vi "_make_3d_data2.vi"(11 "mk3d":T1={"Start(GHz)"=786.0, "Stop(GHz) "=954.0, "Step(GHz) "=8.0, "パス"=path "C:/Documents and Settings/?澤佳?/デスクトップ/data/SISmixer/1108-/110825_O501_164-3-4-B1", "最初のファイル名"="", "取得列 Z"=4, "Text line skip"=0, "リングZ"=0, "リングX"=0, "取得列 X"=0} {"リングX" items=["IF(GHz)", "V(mV)"]; "リングZ" items=["Trx(K)", "I (mA)", "P_PM (dBm)", "P_SP(dBm)", "SBR (dB)", "POUT(dBm/100MHz)", "P-P(dB)"]}) -> (3 "出力ファイル名":string="IV-TRx__matrix_data40_110_110824_O501_164-3-4-B1m.csv.png")   [LabVIEW 2017]
uses:
  <vilib>/Utility/file.llb/Read From Spreadsheet File (string).vi
  <vilib>/Utility/file.llb/Write To Spreadsheet File (DBL).vi
  <vilib>/express/express arith-compare/Formula/XNode/ExpressFormulaBlockNode.xnode
panel:
  out "配列 2":dbl[][](array[numeric])=[[0.0, -0.021515, 0.021133, 0.072174, 0.118256, 0.166397, 0.216446, 0.26619, 0.316162, 0.365219, 0.412979, 0.462189, 0.510864, 0.56633, 0.610428, 0.660324, 0.711594, 0.765305, 0.81337, 0.85968, 0.909805, 0.960464, 1.009, 1.058, 1.125, 1.162, 1.21, 1.26, 1.309, 1.356, 1.412, 1.462, 1.515, 1.567, 1.616, 1.659, 1.711, 1.761, 1.81, 1.858, 1.911, 1.959, 2.009, 2.058, 2.114, 2.159, 2.211, 2.261, 2.316, 2.361, 2.408, 2.456, 2.505, 2.543, 2.576, 2.63, 2.68, 2.75, 2.809, 2.858, 2.912, 2.959, 3.009, 3.063, 3.118, 3.158, 3.208, 3.26, 3.312, 3.358, 3.408, 3.456], [0.0, -2.759, 0.949097, 1.77, 2.716, 3.891, 4.715, 4.971, 5.508, 5.536, 6.039, 6.192, 6.519, 7.303, 7.278, 7.269, 7.129, 7.376, 7.846, 7.675, 7.837, 7.706, 8.182, 8.075, 8.951, 8.67, 8.627, 8.762, 9.293, 9.412, 10.156, 10.516, 10.919, 10.989, 13.586, 11.472, 11.914, 11.996, 12.283, 12.628, 12.357, 12.534, 13.037, 13.245, 12.537, 15.952, 14.566, 14.828, 15.811, 16.809, 17.337, 19.51, 25.082, 46.259, 95.831, 183.994, 262.131, 277.545, 282.7, 286.295, 289.304, 293.353, 297.006, 301.584, 306.857, 311.581, 315.21, 320.633, 325.778, 330.511, 336.539, 341.284], [0.0, -0.024796, 0.014496, 0.070648, 0.117722, 0.16922, 0.21492, 0.268326, 0.313416, 0.36438, 0.413513, 0.462646, 0.50354, 0.561981, 0.611191, 0.662842, 0.711517, 0.765381, 0.815582, 0.861969, 0.909119, 0.95932, 1.012, 1.055, 1.111, 1.16, 1.212, 1.257, 1.312, 1.359, 1.41, 1.46, 1.516, 1.585, 1.615, 1.661, 1.712, 1.76, 1.81, 1.858, 1.912, 1.959, 2.009, 2.056, 2.117, 2.159, 2.211, 2.257, 2.315, 2.36, 2.412, 2.457, 2.506, 2.542, 2.579, 2.621, 2.683, 2.75, 2.807, 2.854, 2.91, 2.96, 3.01, 3.061, 3.119, 3.168, 3.21, 3.26, 3.308, 3.357, 3.409, 3.459], [0.0, -3.03, -0.485229, 2.176, 2.954, 4.175, 4.663, 4.852, 5.463, 5.704, 5.875, 6.094, 6.351, 6.937, 6.775, 7.181, 7.242, 8.023, 7.538, 7.535, 7.892, 7.913, 9.131, 9.052, 7.916, 8.554, 8.661, 8.954, 9.329, 9.561, 10.172, 10.565, 10.916, 11.685, 10.901, 11.368, 11.713, 11.697, 11.792, 12.274, 12.714, 12.448, 12.659, 11.96, 13.339, 14.093, 14.365, 14.911, 15.134, 16.608, 17.584, 19.22, 24.85, 45.2, 92.975, 180.786, 262.372, 277.557, 282.654, 286.032, 289.508, 293.164, 297.324, 301.791, 306.183, 313.147, 315.915, 320.572, 325.543, 331.009, 335.779, 341.519], [0.0, -27.782, -27.509, -29.831, -30.166, -29.882, -28.631, -28.059, -27.897, -27.987, -28.03, -28.065, -27.894, -27.883, -27.792, -27.707, -27.619, -27.792, -27.859, -27.648, -27.37, -27.164, -27.236, -27.394, -27.417, -27.784, -28.542, -29.174, -29.587, -29.571, -29.224, -28.128, -27.366, -26.908, -26.869, -26.719, -26.736, -26.695, -26.838, -26.814, -26.894, -26.348, -26.722, -26.212, -27.382, -27.686, -28.04, -28.527, -29.379, -29.979, -30.586, -31.535, -31.921, -31.348, -31.463, -31.376, -31.686, -30.693, -28.887, -28.036, -28.149, -28.582, -28.835, -28.902, -29.247, -29.316, -29.396, -29.27, -29.234, -29.183, -29.27, -29.233], [0.0, -27.853, -27.485, -29.964, -30.242, -29.717, -28.74, -27.99, -27.882, -28.019, -27.992, -28.197, -27.874, -27.821, -27.809, -27.741, -27.682, -27.792, -27.834, -27.657, -27.449, -27.285, -27.255, -27.421, -27.545, -27.779, -28.486, -29.17, -29.811, -30.056, -29.474, -28.54, -27.809, -27.477, -27.297, -27.124, -27.187, -27.217, -27.343, -27.378, -27.574, -26.883, -27.179, -26.729, -27.946, -28.387, -28.588, -28.94, -29.945, -30.284, -30.987, -31.769, -31.705, -31.834, -31.129, -31.0, -31.339, -30.359, -28.886, -28.164, -28.369, -28.632, -28.643, -28.957, -29.154, -29.248, -29.247, -29.318, -29.311, -29.24, -29.322, -29.566], [0.0, 10000.0, 0.0, 7029.0, 10000.0, 0.0, 8633.0, 0.0, 0.0, 10000.0, 0.0, 7113.0, 0.0, 0.0, 10000.0, 10000.0, 10000.0, 10000.0, 0.0, 10000.0, 10000.0, 7792.0, 10000.0, 10000.0, 7334.0, 0.0, 0.0, 0.0, 4110.0, 1801.0, 3669.0, 2155.0, 1989.0, 1508.0, 2069.0, 2196.0, 1951.0, 1663.0, 1724.0, 1524.0, 1232.0, 1618.0, 1923.0, 1679.0, 1523.0, 1190.0, 1574.0, 2145.0, 1520.0, 2974.0, 2219.0, 3933.0, 0.0, 1800.0, 0.0, 0.0, 0.0, 0.0, 0.0, 7289.0, 4197.0, 10000.0, 0.0, 10000.0, 0.0, 0.0, 0.0, 10000.0, 10000.0, 10000.0, 10000.0, 2710.0], [0.0, 0.0, 0.05, 0.1, 0.15, 0.2, 0.25, 0.3, 0.35, 0.4, 0.45, 0.5, 0.55, 0.6, 0.65, 0.7, 0.75, 0.8, 0.85, 0.9, 0.95, 1.0, 1.05, 1.1, 1.15, 1.2, 1.25, 1.3, 1.35, 1.4, 1.45, 1.5, 1.55, 1.6, 1.65, 1.7, 1.75, 1.8, 1.85, 1.9, 1.95, 2.0, 2.05, 2.1, 2.15, 2.2, 2.25, 2.3, 2.35, 2.4, 2.45, 2.5, 2.55, 2.6, 2.65, 2.7, 2.75, 2.8, 2.85, 2.9, 2.95, 3.0, 3.05, 3.1, 3.15, 3.2, 3.25, 3.3, 3.35, 3.4, 3.45, 3.5]]
  in  "タブ制御器":enum32{"SP ファイル", "YIG関係"}(tab)
  in  "配列 X":T2(array[cluster])=[{"Y label"="IF(GHz)", "Y  range [min:max] "="[3.5:12.5]"}, {"Y label"="V  (mV)", "Y  range [min:max] "="[0:3]"}, {"Y label"="Vg (V)", "Y  range [min:max] "="[0:4]"}, {"Y label"="", "Y  range [min:max] "=""}]
  in  "配列 Z":T3(array[cluster])=[{"Z label"="Trx (K)", "Z  range [min:max] "="[0:500]", "contour  param(start,step,stop) "="200,25,300"}, {"Z label"="I  (mA)", "Z  range [min:max] "="[0:300]", "contour  param(start,step,stop) "="0,10,300"}, {"Z label"="P (dBm)", "Z  range [min:max] "="[-30:-10]", "contour  param(start,step,stop) "="-30,1,-10"}, {"Z label"="P(dBm)", "Z  range [min:max] "="[-60:-40]", "contour  param(start,step,stop) "="-60,5,-40"}, {"Z label"="SBR (dB)", "Z  range [min:max] "="[-2:2]", "contour  param(start,step,stop) "="-3,1,3"}, {"Z label"="Pout (dBm/100MHz)", "Z  range [min:max] "="[-60:-40]", "contour  param(start,step,stop) "="-60,2,-40"}, {"Z label"="PP (dB)", "Z  range [min:max] "="[0:5]", "contour  param(start,step,stop) "="0,1,5"}]
  in  "gnuplotのパス":string="C:\\wintool\\gnuplot\\bin\\wgnuplot.exe  "
  in  "Soption (b:bottom s:surface t:top))":string="sb"
  in  "y  range[min:max]":string="[780:960]"
  in  "y label":string="LO (GHz)"
  out "配列":dbl[][](array[numeric])=[[0.0, 0.0, 0.0, 0.0, 0.0, 0.0, 0.0, 0.0, 0.0, 0.0, 0.0, 0.0, 0.0, 0.0, 0.0, 0.0, 0.0, 0.0, 0.0, 0.0, 0.0, 0.0, 0.0, 0.0, 0.0], [-30.052, -29.746, -29.814, -29.969, -29.665, -29.662, -28.995, -29.934, -30.166, -28.878, -29.619, -29.495, -29.613, -29.184, -28.402, -29.501, -28.588, -28.796, -28.742, -28.754, -28.339, -28.165, -28.518, -27.55, -27.782], [-29.027, -28.715, -29.153, -29.409, -28.957, -29.033, -28.252, -29.414, -29.542, -28.472, -28.837, -28.831, -29.105, -28.292, -27.806, -28.872, -28.1, -28.123, -28.085, -27.916, -27.924, -27.581, -27.997, -27.21, -27.509], [-30.39, -30.323, -30.61, -30.514, -30.678, -30.654, -30.446, -30.508, -30.773, -30.427, -30.544, -30.65, -30.828, -30.482, -30.144, -30.751, -30.552, -30.361, -30.39, -30.146, -30.34, -30.09, -30.3, -29.667, -29.831], [-29.941, -30.022, -30.034, -30.152, -30.317, -30.094, -30.247, -29.872, -30.239, -30.155, -30.317, -30.36, -30.161, -30.262, -30.274, -30.45, -30.369, -30.538, -30.387, -30.182, -30.194, -30.301, -30.351, -30.318, -30.166], [-28.925, -29.309, -29.101, -29.024, -29.103, -29.316, -29.286, -29.285, -29.12, -29.296, -29.419, -29.231, -29.206, -29.34, -29.929, -29.347, -29.672, -29.324, -29.631, -29.465, -29.709, -29.809, -29.655, -29.951, -29.882], [-27.534, -27.559, -27.511, -27.483, -27.798, -27.794, -27.95, -27.71, -27.643, -28.116, -27.783, -28.156, -27.971, -28.202, -28.349, -28.001, -28.379, -28.279, -28.292, -28.389, -28.395, -28.661, -28.371, -28.745, -28.631], [-26.036, -26.401, -26.124, -26.16, -26.51, -26.709, -26.965, -26.46, -26.442, -27.173, -26.796, -26.837, -26.903, -27.301, -27.705, -26.97, -27.513, -27.389, -27.423, -27.39, -27.429, -27.905, -27.423, -28.067, -28.059], [-25.829, -26.185, -25.986, -25.886, -26.231, -26.422, -26.794, -26.247, -26.126, -26.991, -26.688, -26.759, -26.603, -27.026, -27.613, -26.914, -27.266, -27.28, -27.337, -27.27, -27.296, -27.659, -27.438, -27.889, -27.897], [-26.711, -26.496, -26.21, -25.972, -26.228, -26.532, -26.853, -26.326, -26.339, -27.059, -26.765, -26.9, -26.796, -27.158, -27.589, -26.921, -27.433, -27.338, -27.443, -27.274, -27.496, -27.778, -27.462, -28.052, -27.987], [-28.336, -27.383, -26.586, -26.145, -26.328, -26.356, -26.898, -26.354, -26.401, -27.037, -26.97, -27.006, -26.848, -27.248, -27.617, -27.031, -27.525, -27.393, -27.36, -27.493, -27.639, -27.937, -27.571, -28.159, -28.03], [-30.165, -29.108, -27.819, -26.759, -26.475, -26.453, -26.784, -26.296, -26.33, -26.843, -26.885, -26.938, -26.875, -27.147, -27.536, -26.999, -27.437, -27.452, -27.364, -27.453, -27.545, -27.76, -27.662, -28.081, -28.065], [-31.108, -30.641, -29.672, -28.14, -27.396, -26.804, -26.822, -26.039, -25.963, -26.847, -26.635, -26.742, -26.702, -27.062, -27.54, -26.868, -27.324, -27.242, -27.31, -27.289, -27.472, -27.718, -27.466, -27.959, -27.894], [-31.325, -30.996, -30.956, -29.909, -29.093, -27.988, -27.362, -26.275, -25.974, -26.651, -26.392, -26.567, -26.474, -26.867, -27.365, -26.889, -27.282, -27.227, -27.151, -27.316, -27.235, -27.651, -27.325, -28.021, -27.883], [-31.412, -31.069, -31.373, -31.118, -30.681, -29.401, -28.533, -27.065, -26.318, -26.605, -26.309, -26.359, -26.346, -26.885, -27.277, -26.875, -27.221, -27.212, -27.162, -27.382, -27.401, -27.743, -27.438, -28.015, -27.792], [-30.967, -30.611, -31.231, -31.187, -31.083, -30.705, -29.909, -28.673, -27.485, -27.162, -26.405, -26.331, -26.139, -26.754, -27.254, -26.522, -27.073, -26.95, -27.023, -27.286, -27.205, -27.585, -27.151, -27.759, -27.707], [-29.319, -29.132, -30.486, -31.118, -31.272, -30.953, -30.799, -30.484, -29.437, -28.393, -27.325, -26.678, -26.139, -26.547, -26.971, -26.343, -27.044, -26.907, -27.049, -27.026, -27.061, -27.487, -27.211, -27.628, -27.619], [-25.859, -25.949, -28.933, -30.41, -30.719, -30.785, -30.521, -31.094, -30.929, -30.026, -29.03, -27.819, -26.848, -26.761, -27.209, -26.312, -26.979, -26.929, -27.14, -27.044, -27.072, -27.568, -27.147, -27.789, -27.792], [-23.216, -23.364, -25.847, -28.513, -29.447, -30.092, -30.167, -31.357, -31.281, -30.678, -30.457, -29.517, -28.296, -27.578, -27.369, -26.288, -26.829, -26.848, -26.988, -26.902, -27.057, -27.483, -27.23, -27.712, -27.859], [-21.711, -21.945, -23.172, -25.227, -26.494, -28.242, -29.043, -30.591, -30.863, -30.496, -30.873, -30.705, -29.92, -28.783, -27.95, -26.974, -27.08, -26.783, -26.84, -26.743, -26.797, -27.392, -27.132, -27.67, -27.648], [-20.971, -21.049, -21.697, -22.569, -23.665, -25.283, -26.572, -29.538, -30.6, -29.948, -30.859, -30.695, -30.815, -30.164, -28.96, -28.084, -27.386, -26.776, -26.464, -26.475, -26.715, -27.119, -26.614, -27.34, -27.37], [-20.583, -20.627, -20.962, -21.227, -22.06, -23.047, -24.245, -26.961, -29.047, -28.739, -29.93, -30.454, -30.897, -30.617, -29.872, -29.634, -28.43, -27.381, -26.924, -26.542, -26.57, -26.91, -26.647, -27.161, -27.164], [-20.433, -20.452, -20.536, -20.617, -21.398, -21.985, -23.16, -24.206, -26.2, -26.569, -28.59, -29.819, -30.51, -30.435, -30.102, -30.559, -29.75, -28.925, -27.919, -27.165, -26.925, -27.067, -26.591, -27.348, -27.236], [-20.366, -20.511, -20.369, -20.338, -21.079, -21.599, -22.671, -22.605, -23.552, -24.46, -26.343, -28.01, -29.524, -29.89, -29.7, -30.778, -30.152, -29.893, -29.26, -28.387, -27.664, -27.515, -26.778, -27.522, -27.394], [-20.363, -20.627, -20.338, -20.143, -20.962, -21.374, -22.488, -21.838, -22.216, -23.312, -24.254, -25.605, -27.583, -28.582, -29.077, -30.509, -30.117, -30.244, -30.155, -29.578, -28.756, -28.179, -27.387, -27.712, -27.417], [-20.435, -20.825, -20.311, -20.117, -20.964, -21.477, -22.396, -21.519, -21.61, -22.801, -23.226, -24.083, -25.373, -26.648, -27.886, -29.56, -29.485, -30.026, -30.2, -30.129, -29.841, -29.112, -28.515, -28.03, -27.784], [-20.498, -20.976, -20.46, -20.117, -21.038, -21.488, -22.367, -21.389, -21.393, -22.725, -22.802, -23.402, -24.142, -25.318, -26.746, -27.998, -28.544, -29.255, -29.776, -30.089, -30.127, -29.653, -29.528, -28.862, -28.542], [-20.526, -21.12, -20.672, -20.161, -21.115, -21.543, -22.462, -21.285, -21.239, -22.834, -22.679, -23.196, -23.513, -24.763, -26.247, -26.287, -27.312, -28.09, -28.952, -29.591, -29.779, -29.761, -30.116, -29.275, -29.174], [-20.526, -21.195, -20.828, -20.172, -21.172, -21.6, -22.471, -21.218, -21.094, -22.887, -22.554, -23.044, -23.241, -24.482, -26.007, -25.214, -26.256, -26.773, -27.478, -28.714, -29.192, -29.445, -30.063, -29.539, -29.587], [-20.411, -21.054, -20.713, -20.037, -21.083, -21.471, -22.307, -21.055, -20.947, -22.743, -22.443, -22.887, -22.95, -24.288, -25.801, -24.69, -25.799, -25.819, -26.348, -27.278, -28.158, -28.785, -29.554, -29.369, -29.571], [-20.127, -20.603, -20.392, -19.784, -20.822, -21.094, -22.013, -20.769, -20.628, -22.398, -22.228, -22.424, -22.596, -23.827, -25.329, -24.081, -25.208, -25.207, -25.414, -25.966, -26.715, -27.748, -28.459, -28.699, -29.224], [-19.678, -20.088, -20.006, -19.483, -20.542, -20.599, -21.759, -20.493, -20.327, -22.043, -21.824, -22.004, -22.199, -23.307, -24.631, -23.64, -24.651, -24.619, -24.745, -25.033, -25.528, -26.566, -26.85, -27.583, -28.128], [-19.191, -19.754, -19.498, -19.145, -20.308, -20.409, -21.717, -20.302, -20.167, -21.831, -21.632, -21.833, -22.039, -23.151, -24.571, -23.376, -24.347, -24.391, -24.329, -24.689, -25.082, -26.093, -25.949, -27.073, -27.366], [-19.211, -19.714, -19.252, -18.813, -19.997, -20.229, -21.659, -20.195, -20.061, -21.72, -21.552, -21.789, -21.95, -23.107, -24.504, -23.355, -24.342, -24.273, -24.239, -24.681, -25.023, -25.987, -25.632, -26.818, -26.908], [-19.795, -20.015, -19.442, -18.889, -19.74, -20.052, -21.331, -19.946, -19.894, -21.509, -21.444, -21.785, -21.857, -23.097, -24.474, -23.218, -24.263, -24.254, -24.232, -24.569, -24.95, -25.919, -25.413, -26.808, -26.869], [-19.449, -20.177, -19.658, -19.276, -20.155, -20.289, -21.097, -19.775, -19.623, -21.32, -21.173, -21.666, -21.769, -23.081, -24.498, -23.206, -24.251, -24.173, -24.179, -24.575, -24.799, -25.948, -25.273, -26.753, -26.719], [-18.949, -19.943, -19.35, -19.074, -20.276, -20.89, -21.656, -20.131, -19.804, -21.129, -20.872, -21.35, -21.514, -22.923, -24.582, -23.123, -24.253, -24.248, -24.181, -24.538, -24.737, -25.933, -25.249, -26.733, -26.736], [-19.162, -20.06, -19.267, -18.709, -19.791, -20.411, -21.267, -20.255, -20.189, -21.766, -21.245, -21.29, -21.296, -22.484, -24.331, -22.949, -24.303, -24.177, -24.253, -24.478, -24.805, -25.998, -25.237, -26.757, -26.695], [-19.515, -20.359, -19.713, -18.892, -19.951, -20.381, -21.096, -19.817, -19.739, -21.545, -21.464, -22.098, -21.982, -22.673, -23.807, -22.544, -23.892, -23.981, -24.2, -24.474, -24.709, -26.001, -25.244, -26.815, -26.838], [-19.68, -20.533, -20.021, -19.209, -20.278, -20.705, -21.446, -19.933, -19.647, -21.432, -21.03, -21.367, -21.66, -23.098, -24.98, -23.242, -23.809, -23.462, -23.618, -24.078, -24.667, -25.886, -25.353, -26.853, -26.814], [-19.78, -20.586, -20.135, -19.388, -20.481, -20.887, -21.749, -20.252, -19.932, -21.971, -21.5, -21.587, -21.625, -22.627, -23.935, -22.767, -24.12, -24.687, -24.509, -24.061, -24.117, -25.34, -25.133, -26.873, -26.894], [-19.869, -20.378, -20.18, -19.485, -20.619, -20.844, -21.974, -20.446, -20.217, -22.224, -21.887, -21.97, -22.027, -23.204, -24.648, -22.924, -23.943, -23.686, -23.72, -24.291, -25.336, -25.973, -24.853, -26.153, -26.348], [-20.034, -20.552, -20.229, -19.644, -20.783, -20.945, -22.328, -20.643, -20.373, -22.349, -22.091, -22.195, -22.285, -23.563, -24.936, -23.403, -24.618, -24.403, -24.226, -24.219, -24.385, -25.248, -25.259, -27.29, -26.722], [-20.245, -20.842, -20.355, -19.797, -21.028, -21.137, -22.642, -20.868, -20.587, -22.529, -22.294, -22.444, -22.517, -23.728, -25.143, -23.757, -24.854, -24.839, -24.724, -24.994, -25.28, -26.184, -25.297, -26.75, -26.212], [-20.506, -21.291, -20.662, -20.084, -21.327, -21.531, -22.883, -21.149, -20.887, -22.594, -22.555, -22.735, -22.766, -24.068, -25.432, -24.023, -25.105, -25.042, -24.966, -25.295, -25.655, -26.834, -26.063, -27.47, -27.382], [-20.844, -21.734, -20.971, -20.424, -21.678, -21.983, -23.233, -21.514, -21.227, -22.961, -22.715, -23.082, -23.063, -24.379, -25.745, -24.277, -25.422, -25.441, -25.294, -25.656, -25.882, -26.952, -26.255, -27.789, -27.686], [-21.425, -22.457, -21.525, -20.972, -22.263, -22.771, -23.714, -22.035, -21.75, -23.513, -23.321, -23.584, -23.55, -24.773, -26.259, -24.751, -25.911, -25.918, -25.673, -26.092, -26.282, -27.276, -26.562, -28.177, -28.04], [-22.235, -23.182, -22.342, -21.737, -23.033, -23.393, -24.23, -22.763, -22.501, -24.284, -23.861, -24.291, -24.239, -25.466, -26.932, -25.315, -26.552, -26.34, -26.363, -26.614, -26.679, -27.815, -27.241, -28.599, -28.527], [-23.615, -24.333, -23.826, -23.011, -24.267, -24.621, -25.386, -23.97, -23.769, -25.471, -25.055, -25.442, -25.385, -26.401, -27.751, -26.275, -27.247, -27.338, -27.272, -27.434, -27.685, -28.583, -28.052, -29.296, -29.379], [-25.259, -25.824, -25.476, -24.8, -25.771, -26.047, -26.63, -25.349, -25.362, -26.868, -26.38, -26.692, -26.728, -27.668, -28.755, -27.498, -28.514, -28.416, -28.316, -28.46, -28.581, -29.369, -28.905, -29.857, -29.979], [-27.848, -27.914, -28.011, -27.447, -27.945, -27.974, -28.493, -27.918, -27.774, -28.656, -28.381, -28.594, -28.649, -29.418, -29.906, -29.138, -29.724, -29.416, -29.786, -29.634, -29.905, -30.401, -29.999, -30.732, -30.586], [-30.866, -30.48, -30.557, -30.384, -30.543, -30.528, -30.866, -30.593, -30.305, -30.495, -30.707, -30.707, -30.969, -30.948, -31.045, -30.753, -30.928, -31.199, -31.089, -31.223, -30.877, -31.361, -31.215, -31.541, -31.535], [-31.681, -31.758, -31.449, -31.609, -31.544, -31.613, -31.486, -31.386, -31.644, -31.593, -31.576, -31.54, -31.63, -31.668, -31.643, -31.693, -31.783, -31.539, -31.469, -31.582, -31.822, -31.641, -31.806, -31.573, -31.921], [-31.231, -31.504, -31.174, -31.45, -31.508, -31.612, -31.653, -31.566, -31.43, -31.574, -31.564, -31.526, -31.392, -31.342, -31.365, -31.338, -31.676, -31.357, -31.362, -31.233, -31.452, -31.447, -31.334, -31.61, -31.348], [-31.542, -31.379, -31.49, -31.343, -31.329, -31.083, -31.713, -31.209, -31.499, -31.749, -31.493, -31.202, -31.436, -31.485, -31.507, -31.527, -31.304, -31.329, -31.396, -31.495, -31.354, -31.585, -31.561, -31.432, -31.463], [-31.459, -31.686, -31.46, -31.591, -31.301, -31.524, -31.421, -31.505, -31.404, -31.463, -31.181, -31.356, -31.494, -31.573, -31.376, -31.395, -31.449, -31.403, -31.612, -31.51, -31.155, -31.531, -31.35, -31.327, -31.376], [-31.201, -31.316, -31.242, -31.249, -31.338, -31.267, -31.298, -31.258, -31.323, -31.549, -31.374, -31.349, -31.236, -31.258, -31.263, -31.121, -31.479, -31.361, -31.511, -31.399, -31.106, -31.232, -31.423, -31.424, -31.686], [-30.224, -30.409, -30.232, -30.077, -30.311, -30.444, -30.518, -30.376, -30.258, -30.306, -30.381, -30.515, -30.501, -30.653, -30.641, -30.253, -30.59, -30.683, -30.362, -30.289, -30.48, -30.648, -30.62, -30.91, -30.693], [-28.71, -28.767, -28.534, -28.623, -28.769, -28.619, -28.83, -28.745, -28.651, -28.737, -28.738, -28.723, -28.592, -28.897, -28.801, -28.737, -28.918, -28.901, -28.915, -28.864, -28.843, -28.817, -28.893, -28.892, -28.887], [-28.052, -28.055, -27.961, -27.985, -28.062, -28.097, -27.99, -28.119, -28.17, -28.098, -28.095, -28.07, -28.245, -28.054, -28.159, -28.164, -28.064, -28.057, -28.012, -28.095, -28.038, -28.156, -28.189, -28.06, -28.036], [-28.257, -28.161, -28.169, -28.257, -28.171, -28.161, -28.322, -28.28, -28.36, -28.289, -28.248, -28.302, -28.33, -28.179, -28.321, -28.354, -28.198, -28.261, -28.219, -28.18, -28.269, -28.221, -28.259, -28.161, -28.149], [-28.525, -28.539, -28.595, -28.534, -28.579, -28.481, -28.424, -28.603, -28.548, -28.469, -28.463, -28.555, -28.546, -28.432, -28.501, -28.525, -28.552, -28.543, -28.459, -28.51, -28.509, -28.586, -28.503, -28.503, -28.582], [-28.635, -28.743, -28.739, -28.771, -28.647, -28.757, -28.83, -28.735, -28.658, -28.765, -28.834, -28.739, -28.846, -28.759, -28.829, -28.844, -28.891, -28.799, -28.734, -28.825, -28.699, -28.791, -28.73, -28.731, -28.835], [-29.115, -28.824, -28.837, -28.918, -28.896, -28.868, -29.045, -28.91, -28.969, -28.984, -28.912, -28.908, -28.998, -28.844, -28.971, -28.959, -28.948, -29.127, -28.883, -29.099, -29.057, -28.931, -28.911, -28.987, -28.902], [-29.237, -29.147, -28.996, -29.107, -28.936, -29.098, -29.127, -29.095, -28.944, -29.119, -29.047, -29.097, -29.07, -29.001, -29.201, -28.966, -29.213, -29.009, -28.951, -29.045, -29.083, -29.149, -29.094, -29.236, -29.247], [-29.405, -29.066, -29.223, -29.198, -29.213, -29.097, -29.059, -29.111, -29.015, -29.045, -29.176, -29.232, -29.079, -29.175, -29.102, -29.144, -29.106, -29.269, -29.229, -29.182, -29.1, -29.15, -29.108, -29.262, -29.316], [-29.053, -29.321, -29.363, -29.24, -29.294, -29.103, -29.188, -29.077, -29.123, -29.185, -29.14, -29.232, -29.431, -29.201, -29.398, -29.301, -29.108, -29.169, -29.186, -29.26, -29.247, -29.248, -29.245, -29.157, -29.396], [-29.193, -29.298, -29.242, -29.261, -29.149, -29.384, -29.365, -29.198, -29.045, -29.324, -29.236, -29.297, -29.225, -29.158, -29.241, -29.198, -29.136, -29.303, -29.258, -29.2, -29.276, -29.304, -29.256, -29.278, -29.27], [-29.286, -29.03, -29.305, -29.25, -29.432, -29.263, -29.291, -29.227, -29.398, -29.146, -29.389, -29.368, -29.179, -29.314, -29.407, -29.365, -29.369, -29.194, -29.498, -29.283, -29.266, -29.358, -29.331, -29.376, -29.234], [-29.438, -29.246, -29.247, -29.376, -29.285, -29.306, -29.402, -29.396, -29.262, -29.08, -29.394, -29.417, -29.094, -29.315, -29.295, -29.325, -29.4, -29.292, -29.133, -29.149, -29.29, -29.368, -29.31, -29.265, -29.183], [-29.163, -29.29, -29.293, -29.278, -29.267, -29.363, -29.199, -29.303, -29.279, -29.293, -29.248, -29.232, -29.344, -29.308, -29.328, -29.259, -29.187, -29.339, -29.347, -29.33, -29.317, -29.213, -29.237, -29.405, -29.27], [-29.035, -29.254, -29.19, -29.264, -29.327, -29.226, -29.276, -29.187, -29.283, -29.296, -29.23, -29.208, -29.024, -29.226, -29.259, -29.309, -29.16, -29.363, -29.297, -29.33, -29.232, -29.214, -29.172, -29.278, -29.233]]
  in  "周波数フォーマット":string="%.1f"
  out "周波数":string="786.0"
  out "接尾語":string="0_140_111002_K105_164-5-3-A1m.csv"
  out "接頭語":string="SP_"
  # "<= Mix通常測定では  %.1f"
  # "IVTrx ファイル\n1:Ihot\n2:Vcold\n3:Icold\n4:Phot\n5:Pcold\n6:Trx"
  # "LP ファイル\n1:volt\n2: current\n3:Phot\n4:Pcold\n5:Trx"
  # "IV ファイル\n1: current\n2:Phot\n3:Pcold"
  # "A_YIG ファイル\nskip1\n\n13:Pout"
  # "SP ファイル\n0:IF\n1：Phot\n2:Pcold \n3:dummy\n4:Trx"
  # "A_SBR ファイル\nskip2\n\n8:TrxDSB\n9:Tmes 1\n10:Tmes 2\n15:SBR 1\n16:SBR 2"
  # "A_YIG ファイル\nskip1\n0: IF\n9: Trx\n12: Pout\n14: PP(2GHz)"
  # "PV_YIG ファイル\nskip0\n0:TS\n1:LO\n\n4:IF\n6:pp(2GHz)"
  # "IFS_YIG ファイル\nskip0\n0:TS\n1:LO\n\n4:IF\n6:IF spectrum"
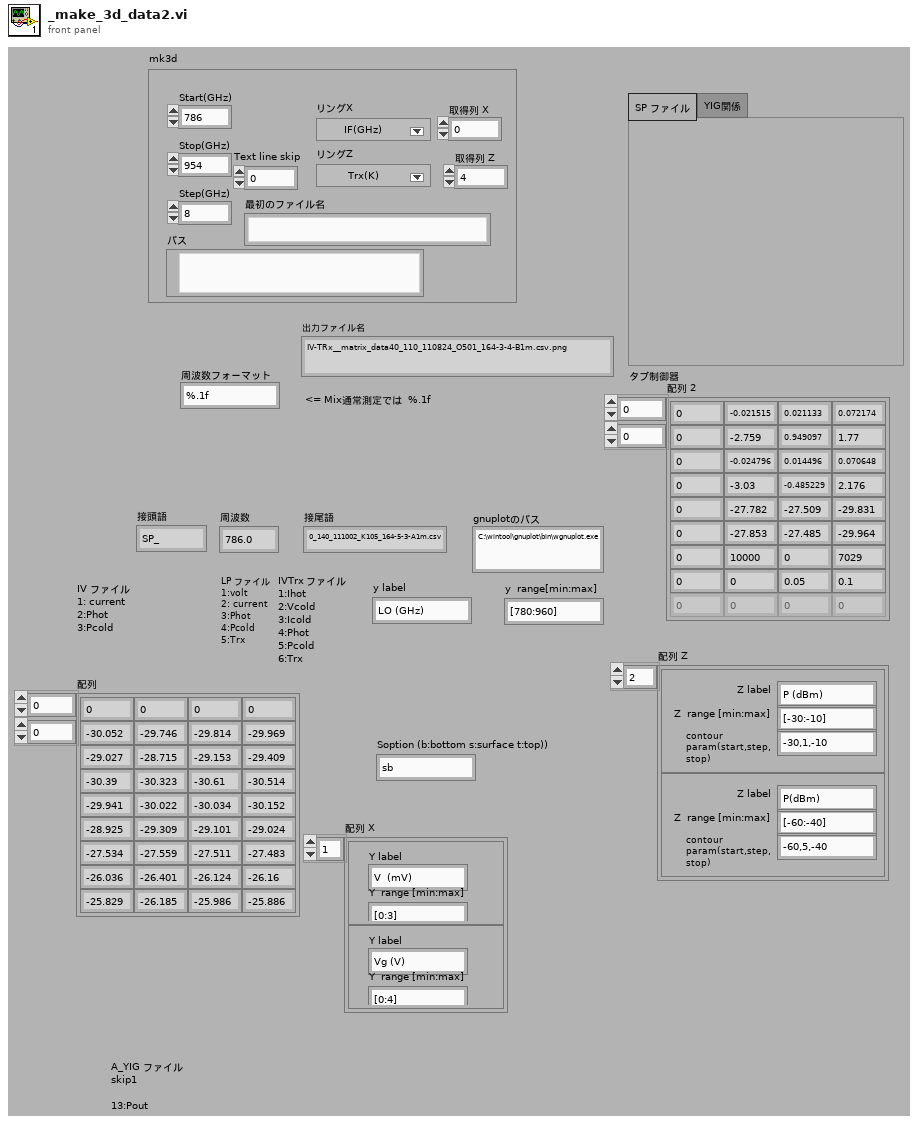
[diagram p1: front panel]
types:
  T1 = cluster{"Start(GHz)":dbl, "Stop(GHz) ":dbl, "Step(GHz) ":dbl, "パス":path, "最初のファイル名":string, "取得列 Z":i32, "Text line skip":i32, "リングZ":u16, "リングX":u16, "取得列 X":i32}
  T2 = cluster{"Y label":string, "Y  range [min:max] ":string}[]
  T3 = cluster{"Z label":string, "Z  range [min:max] ":string, "contour  param(start,step,stop) ":string}[]
  T4 = cluster{"Z label":string, "Z  range [min:max] ":string, "contour  param(start,step,stop) ":string}
  T5 = cluster{"Y label":string, "Y  range [min:max] ":string}
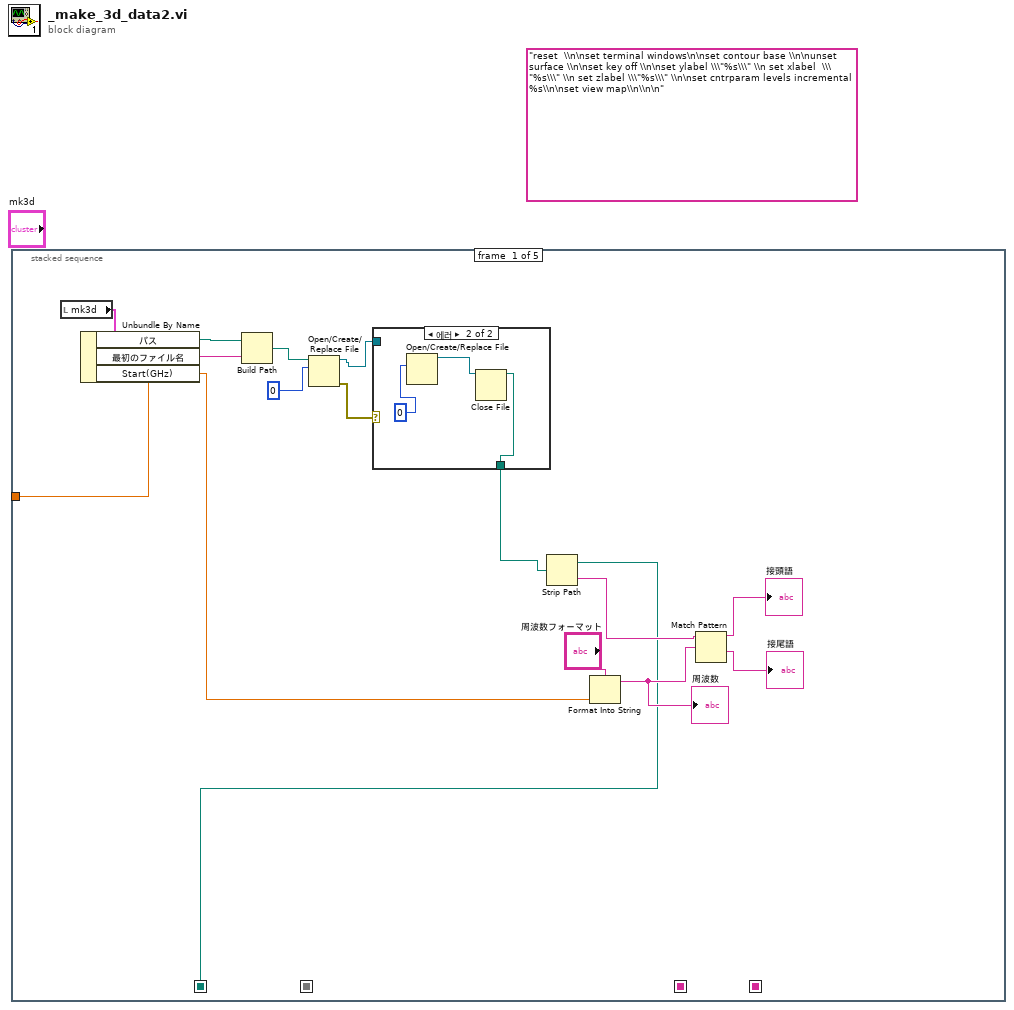
[diagram p0: block diagram]
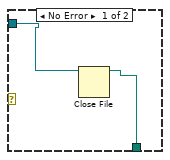
[diagram p2: hidden frame]
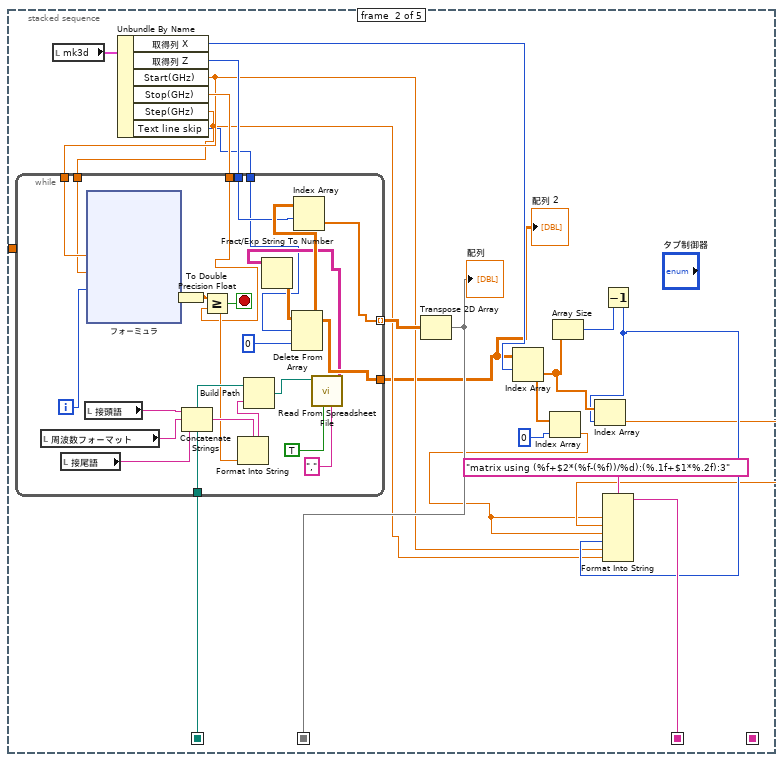
[diagram p3: hidden frame]
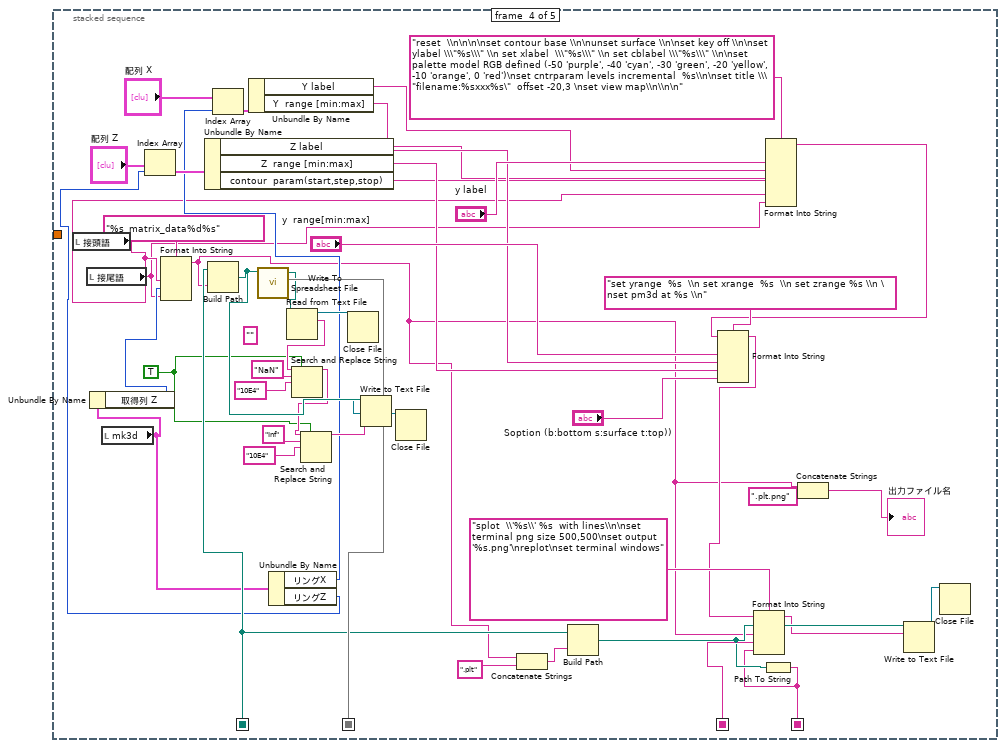
[diagram p5: hidden frame]
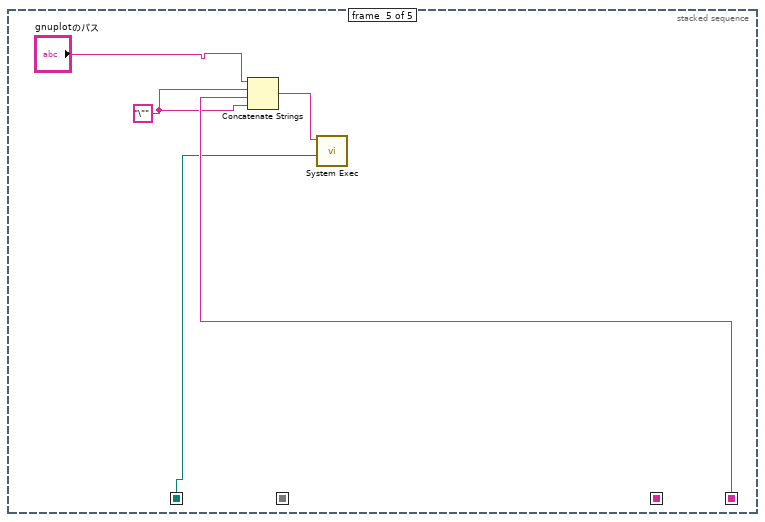
[diagram p6: hidden frame]
diagram:
  (unwired) "reset  \\n\nset terminal windows\n\nset contour base \\n\nunset surface \\n\nset key off \\n\nset ylabel \\\"%s\\\" \\n set xlabel  \\\"%s\\\" \\n set zlabel \\\"%s\\\" \\n\nset cntrparam levels incremental  %s\\n\nset view map\\n\\n\n"
  n1 = stacked-sequence {
    seq-local: [w10 _ _ _ _] -> [_ w39 _ w112 w123]
    seq-local: [_ w38 _ _ _] -> [_ _ _ w121 _]
    seq-local: [_ w34 _ _ _] -> [_ _ _ w119 _]
    seq-local: [_ _ _ w75 _] -> [_ _ _ _ w125]
    tunnel: [w3 _ _ _ _] -> _
    frame #0 {
      n2 = local read "mk3d"() -> (w9:T1)
      n3 = Unbundle By Name(w9) -> ("パス"=w8:path, "最初のファイル名"=w7:string, "Start(GHz)"=w3:dbl)
      n4 = Build Path(base path=w8, name or relative path=w7) -> (appended path=w6:path)
      n5 = Open/Create/Replace File(file path (use dialog)=w6, operation (0:open)=0) -> (refnum out=w2:refnum<file>, error out=w4:errorcluster)  [unwired: 4 in, 1 out]
      n6 = case shown="에러" w4 {
        tunnel: w2 -> [w17 _]
        tunnel: [w16 w18] -> w1
        frame No Error {
          n7 = Close File(refnum=w17) -> (path=w16:path)  [unwired: 1 in, 1 out]
        }
        frame Error {
          n8 = Open/Create/Replace File(operation (0:open)=0) -> (refnum out=w19:refnum<file>)  [unwired: 5 in, 2 out]
          n9 = Close File(refnum=w19) -> (path=w18:path)  [unwired: 1 in, 1 out]
        }
      }
      n10 = Strip Path(path=w1) -> (stripped path=w10:path, name=w14:string)
      n11 = Format Into String(format string="周波数フォーマット", w3) -> (resulting string=w11:string)  [unwired: 2 in, 1 out]
      "周波数" <- w11
      n12 = Match Pattern(string=w14, regular expression=w11) -> (before substring=→"接頭語":string, after substring=→"接尾語":string)  [unwired: 1 in, 2 out]
    }
    frame #1 {
      n13 = local read "mk3d"() -> (w31:T1)
      n14 = Unbundle By Name(w31) -> ("取得列 X"=w25:i32, "取得列 Z"=w30:i32, "Start(GHz)"=w27:dbl, "Stop(GHz)"=w29:dbl, "Step(GHz)"=w26:dbl, "Text line skip"=w22:i32)
      n15 = while {
        tunnel: w39 -> [w59]
        tunnel: [w48] -> w21
        tunnel: [w44] -> w32 mode=indexing
        tunnel: w30 -> [w47]
        tunnel: w27 -> [w43]
        tunnel: w26 -> [w42]
        tunnel: w29 -> [w41]
        tunnel: w22 -> [w40]
        i -> [w62]
        stop <- w60 stop-if-true
        n16 = local read "周波数フォーマット"() -> (w57:string)
        n17 = local read "接尾語"() -> (w56:string)
        n18 = local read "接頭語"() -> (w58:string)
        n19 = xnode "フォーミュラ"("start"=w43, "step"=w42, "i"=w62) -> ("結果"=w61:dbl)  [unwired: 1 in, 1 out]
        n20 = To Double Precision Float(number=w61) -> (double precision float=w54:dbl)
        n21 = Concatenate Strings(w58, w57, w56) -> (w55:string)
        n22 = Greater Or Equal?(x=w54, y=w41) -> (x >= y?=w60:bool)
        n23 = Format Into String(format string=w55, w54) -> (resulting string=w53:string)  [unwired: 2 in, 1 out]
        n24 = Build Path(base path=w59, name or relative path=w53) -> (appended path=w52:path)
        n25 = call-poly <vilib>:"Read From Spreadsheet File.vi"("delimiter (\\t)"=",", "transpose (no:F)"=TRUE, "file path (dialog if empty)"=w52) -> ("all rows"=w46:string[][])  [unwired: 4 in, 4 out]
        n26 = Fract/Exp String To Number(string=w46) -> (number=w45:dbl[][])  [unwired: 3 in, 1 out]
        n27 = Delete From Array(array=w45, length=w40, index (col)=0) -> (array with subset deleted=w48:dbl[][])  [unwired: 1 in, 1 out]
        n28 = Index Array(array=w48, index (row)=w47) -> (element=w44:dbl[])  [unwired: 1 in]
      }
      "配列 2" <- w21
      n29 = Transpose 2D Array(2D array=w32) -> (transposed array=w38:dbl[][])
      "配列" <- w38
      n30 = Index Array(array=w21, index (row)=w25) -> (element=w37:dbl[])  [unwired: 1 in]
      n31 = Index Array(array=w37, index=0) -> (element=w23:dbl)
      n32 = Array Size(array=w37) -> (size(s)=w35:i32)
      n33 = Decrement(x=w35) -> (x-1=w33:i32)
      n34 = Index Array(array=w37, index=w33) -> (element=w28:dbl)
      n35 = Format Into String(format string="matrix using (%f+$2*(%f-(%f))/%d):(%.1f+$1*%.2f):3", w23, w28, w23, w33, w27, w26) -> (resulting string=w34:string)  [unwired: 2 in, 1 out]
    }
    frame #2 {
    }
    frame #3 {
      w97 = TRUE
      (unwired) ""
      n36 = local read "接頭語"() -> (w80:string)
      n37 = local read "接尾語"() -> (w79:string)
      n38 = local read "mk3d"() -> (w86:T1)
      n39 = Unbundle By Name(w86) -> ("取得列 Z"=w87:i32)
      n40 = Format Into String(format string="%s_matrix_data%d%s", w80, w87, w79) -> (resulting string=w76:string)  [unwired: 2 in, 1 out]
      n41 = Build Path(base path=w112, name or relative path=w76) -> (appended path=w104:path)
      n42 = call-poly <vilib>:"Write To Spreadsheet File.vi"("2D data"=w121, "file path (dialog if empty)"=w104) -> ("new file path (Not A Path if cancelled)"=w109:path)  [unwired: 6 in]
      n43 = Unbundle By Name(w86) -> ("リングX"=w85:u16, "リングZ"=w84:u16)
      n44 = Index Array(array="配列 Z", index=w84) -> (element=w94:T4)
      n45 = Unbundle By Name(w94) -> ("Z label"=w89:string, "Z  range [min:max]"=w91:string, "contour  param(start,step,stop)"=w88:string)
      n46 = Index Array(array="配列 X", index=w85) -> (element=w95:T5)
      n47 = Unbundle By Name(w95) -> ("Y label"=w90:string, "Y  range [min:max]"=w92:string)
      n48 = Read from Text File(file (use dialog)=w109) -> (refnum out=w105:refnum<file>, text=w108:string)  [unwired: 3 in, 2 out]
      n49 = Search and Replace String(replace all?=w97, input string=w108, search string="NaN", replace string="10E4") -> (result string=w99:string)  [unwired: 4 in, 3 out]
      n50 = Search and Replace String(replace all?=w97, input string=w99, search string="Inf", replace string="10E4") -> (result string=w98:string)  [unwired: 4 in, 3 out]
      n51 = Close File(refnum=w105) -> ()  [unwired: 1 in, 2 out]
      n52 = Write to Text File(file (use dialog)=w104, text=w98) -> (refnum out=w103:refnum<file>)  [unwired: 2 in, 2 out]
      n53 = Close File(refnum=w103) -> ()  [unwired: 1 in, 2 out]
      n54 = Concatenate Strings(w76, ".plt") -> (w111:string)
      n55 = Build Path(base path=w112, name or relative path=w111) -> (appended path=w110:path)
      n56 = Path To String(path=w110) -> (string=w75:string)
      n57 = Format Into String(format string="reset  \\n\n\n\nset contour base \\n\nunset surface \\n\nset key off \\n\nset ylabel \\\"%s\\\" \\n set xlabel  \\\"%s\\\" \\n set cblabel \\\"%s\\\" \\n\nset palette model RGB defined (-50 'purple', -40 'cyan', -30 'green', -20 'yellow', -10 'orange', 0 'red')\nset cntrparam levels incremental  %s\\n\nset title \\\"filename:%sxxx%s\"  offset -20,3 \nset view map\\n\\n\n", "y label", w90, w89, w88, w80, w79) -> (resulting string=w83:string)  [unwired: 2 in, 1 out]
      n58 = Format Into String(format string="set yrange  %s  \\n set xrange  %s  \\n set zrange %s \\n \nset pm3d at %s \\n", initial string=w83, "y  range[min:max]", w92, w91, "Soption (b:bottom s:surface t:top))") -> (resulting string=w82:string)  [unwired: 1 in, 1 out]
      n59 = Format Into String(format string="splot  \\'%s\\' %s  with lines\\n\nset terminal png size 500,500\nset output '%s.png'\nreplot\nset terminal windows", initial string=w82, w76, w119, w75) -> (resulting string=w81:string)  [unwired: 1 in, 1 out]
      n60 = Concatenate Strings(w76, ".plt.png") -> (→"出力ファイル名":string)
      n61 = Write to Text File(file (use dialog)=w110, text=w81) -> (refnum out=w102:refnum<file>)  [unwired: 2 in, 2 out]
      n62 = Close File(refnum=w102) -> ()  [unwired: 1 in, 2 out]
    }
    frame #4 {
      w124 = "\""
      n63 = Concatenate Strings("gnuplotのパス", w124, w125, w124) -> (w126:string)
      n64 = call <vilib>:"System Exec.vi"("working directory"=w123, "command line"=w126) -> ()  [unwired: 6 in, 4 out]
    }
  }
